vi "SimulatedConfigRefGlobal.vi"() -> ()   [LabVIEW 2017, in "EmsaAcquisition.lvlib"]
uses:
  <vilib>/addons/InsightCM/Devices/Shared/Emsa/EmsaAcquisition/EmsaAcquisition.lvlib
  <vilib>/addons/InsightCM/Devices/Shared/Emsa/EmsaAcquisition/controls/SimulatedConfigRefs.ctl
panel:
  in  "Simulated Config Refs":T1
  in  "Hide UI":bool
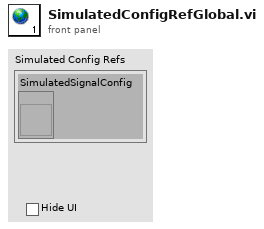
[diagram p1: front panel]
types:
  T1 = typedef "EmsaAcquisition.lvlib/SimulatedConfigRefs.ctl" = cluster{"SimulatedSignalConfig":refnum<vi>}
diagram:
